vi "Set Measurement.vi"(6 "Escala":dbl, 8 "error in (no error)":errorcluster, 9 "Range ON/OFF":bool, 10 "Grandeza Elétrica":string, 11 "Multimeter in":refnum<class "Multimeter.lvclass">) -> (0 "error out":errorcluster, 3 "Multimeter out":refnum<class "Multimeter.lvclass">)   [LabVIEW 2015, in "Multimeter.lvclass"]
uses:
  Multimeter.lvclass
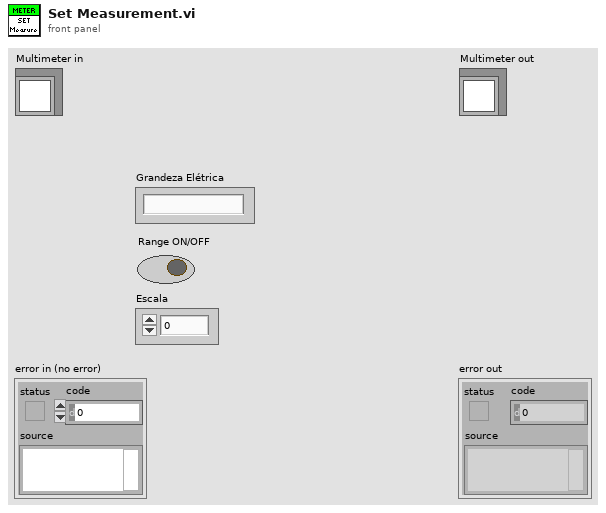
[diagram p1: front panel]
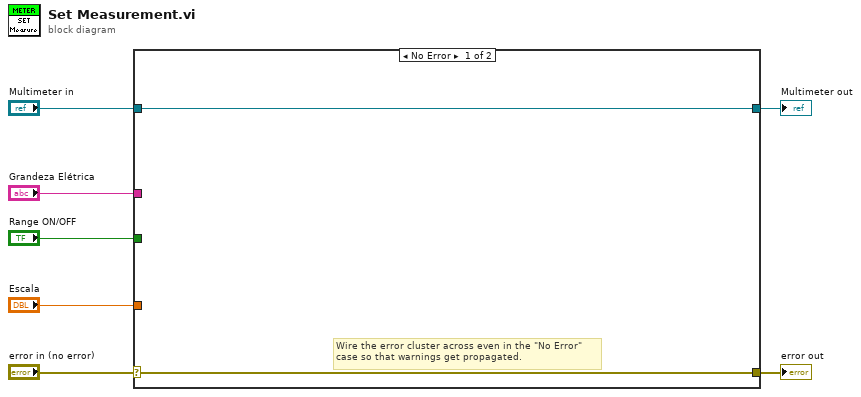
[diagram p0: block diagram]
diagram:
  n1 = case shown="No Error" "error in (no error)" {
    selector: "error in (no error)" -> [w8 w11]
    tunnel: [w8 w11] -> w6
    tunnel: [w9 w10] -> w4
    tunnel: "Multimeter in" -> [w9 w10]
    tunnel: "Grandeza Elétrica" -> [_ _]
    tunnel: "Range ON/OFF" -> [_ _]
    tunnel: "Escala" -> [_ _]
    frame No Error {
      # "Wire the error cluster across even in the \"No Error\"\ncase so that warnings get propagated."
    }
    frame Error {
    }
  }
  "error out" <- w6
  "Multimeter out" <- w4
